vi "ColorCycle.vi"(8 "Error In":errorcluster, 10 "Reset":bool, 11 "Colorcycle":T1(ring)) -> (0 "Error Out":errorcluster, 1 "Color Count":i32, 2 "All Colors":u32[](array[numeric]) format="%x", 3 "Color":u32=16716306 format="%06x")   [LabVIEW 2022 SP3, in "hse-misc.lvlib"]
doc: "With every call, this VI returns a color from a color pallet. If the last color from a pallet is reached, the VI continues with the first color.\n\nThis Vi is useful to give plots and graphs better looking colors.\n\nThe color sets are inspired by a subset of the colormaps from the Python plotting library Matplotlib.\n\n____\nHAMPEL SOFTWARE ENGINEERING v3.8.0 (2023-12-18 14:41)"
uses:
  hse-misc.lvlib
panel:
  out "Color (preview)":u32(colorbox)
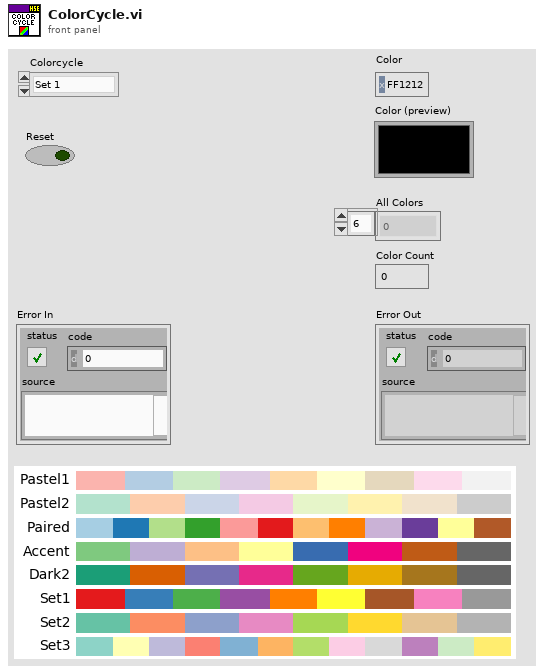
[diagram p1: front panel]
types:
  T1 = enum16{"Set 1", "Set 2", "Set 3", "Pastel 1", "Pastel 2", "Accent", "Dark", "Paired"}
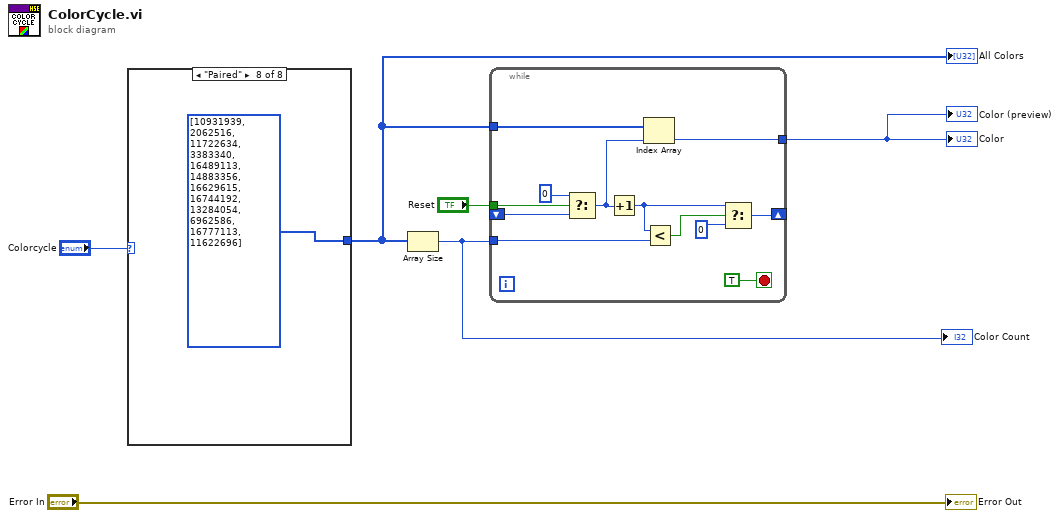
[diagram p0: block diagram]
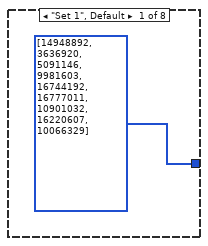
[diagram p2: hidden frame]
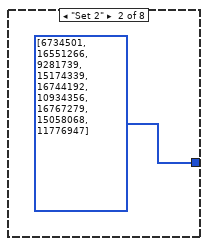
[diagram p3: hidden frame]
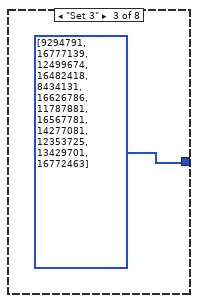
[diagram p4: hidden frame]
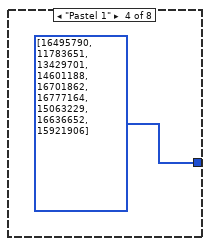
[diagram p5: hidden frame]
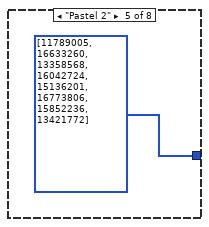
[diagram p6: hidden frame]
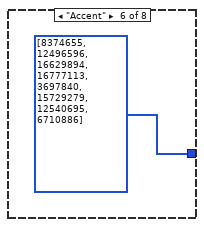
[diagram p7: hidden frame]
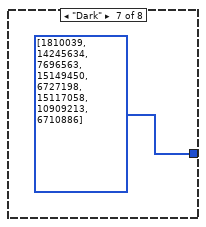
[diagram p8: hidden frame]
diagram:
  n1 = case shown="\"Paired\"" "Colorcycle" {
    tunnel: [u32[] [14948892, 3636920, 5091146, 9981603, 16744192, 16777011, 10901032, 16220607, 10066329] u32[] [6734501, 16551266, 9281739, 15174339, 16744192, 10934356, 16767279, 15058068, 11776947] u32[] [9294791, 16777139, 12499674, 16482418, 8434131, 16626786, 11787881, 16567781, 14277081, 12353725, 13429701, 16772463] u32[] [16495790, 11783651, 13429701, 14601188, 16701862, 16777164, 15063229, 16636652, 15921906] u32[] [11789005, 16633260, 13358568, 16042724, 15136201, 16773806, 15852236, 13421772] u32[] [8374655, 12496596, 16629894, 16777113, 3697840, 15729279, 12540695, 6710886] u32[] [1810039, 14245634, 7696563, 15149450, 6727198, 15117058, 10909213, 6710886] u32[] [10931939, 2062516, 11722634, 3383340, 16489113, 14883356, 16629615, 16744192, 13284054, 6962586, 16777113, 11622696]] -> w3
    frame "Set 1", Default {
    }
    frame "Set 2" {
    }
    frame "Set 3" {
    }
    frame "Pastel 1" {
    }
    frame "Pastel 2" {
    }
    frame "Accent" {
    }
    frame "Dark" {
    }
    frame "Paired" {
    }
  }
  "All Colors" <- w3
  n2 = Array Size(array=w3) -> (size(s)=w4:i32)
  "Color Count" <- w4
  n3 = while {
    shift-right: [w22] -> _
    shift-left: _ -> [w17]
    tunnel: w4 -> [w25]
    tunnel: [w21] -> w1
    tunnel: w3 -> [w20]
    tunnel: "Reset" -> [w16]
    stop <- TRUE stop-if-true
    n4 = Select(t=0, s=w16, f=w17) -> (s? t:f=w18:i32)
    n5 = Increment(x=w18) -> (x+1=w24:i32)
    n6 = Index Array(array=w20, index=w18) -> (element=w21:u32)
    n7 = Less?(x=w24, y=w25) -> (x < y?=w19:bool)
    n8 = Select(t=w24, s=w19, f=0) -> (s? t:f=w22:i32)
  }
  "Color" <- w1
  "Color (preview)" <- w1
  "Error Out" <- "Error In"
